vi "ATF-Graph Screen.vi"() -> ()   [LabVIEW 2022 SP3]
panel:
  in  "Monitor":u16=1
  out "Waveform 6":dbl[][](graph)
  out "Waveform 5":waveform(dbl)[](graph)
  out "Waveform 4":waveform(dbl)[](graph)
  out "Waveform 3":waveform(dbl)[](graph)
  out "Waveform 2":waveform(dbl)[](graph)
  out "Waveform 1":waveform(dbl)[](graph)
  in  "EXIT":bool
  # "GRAPH SCREEN"
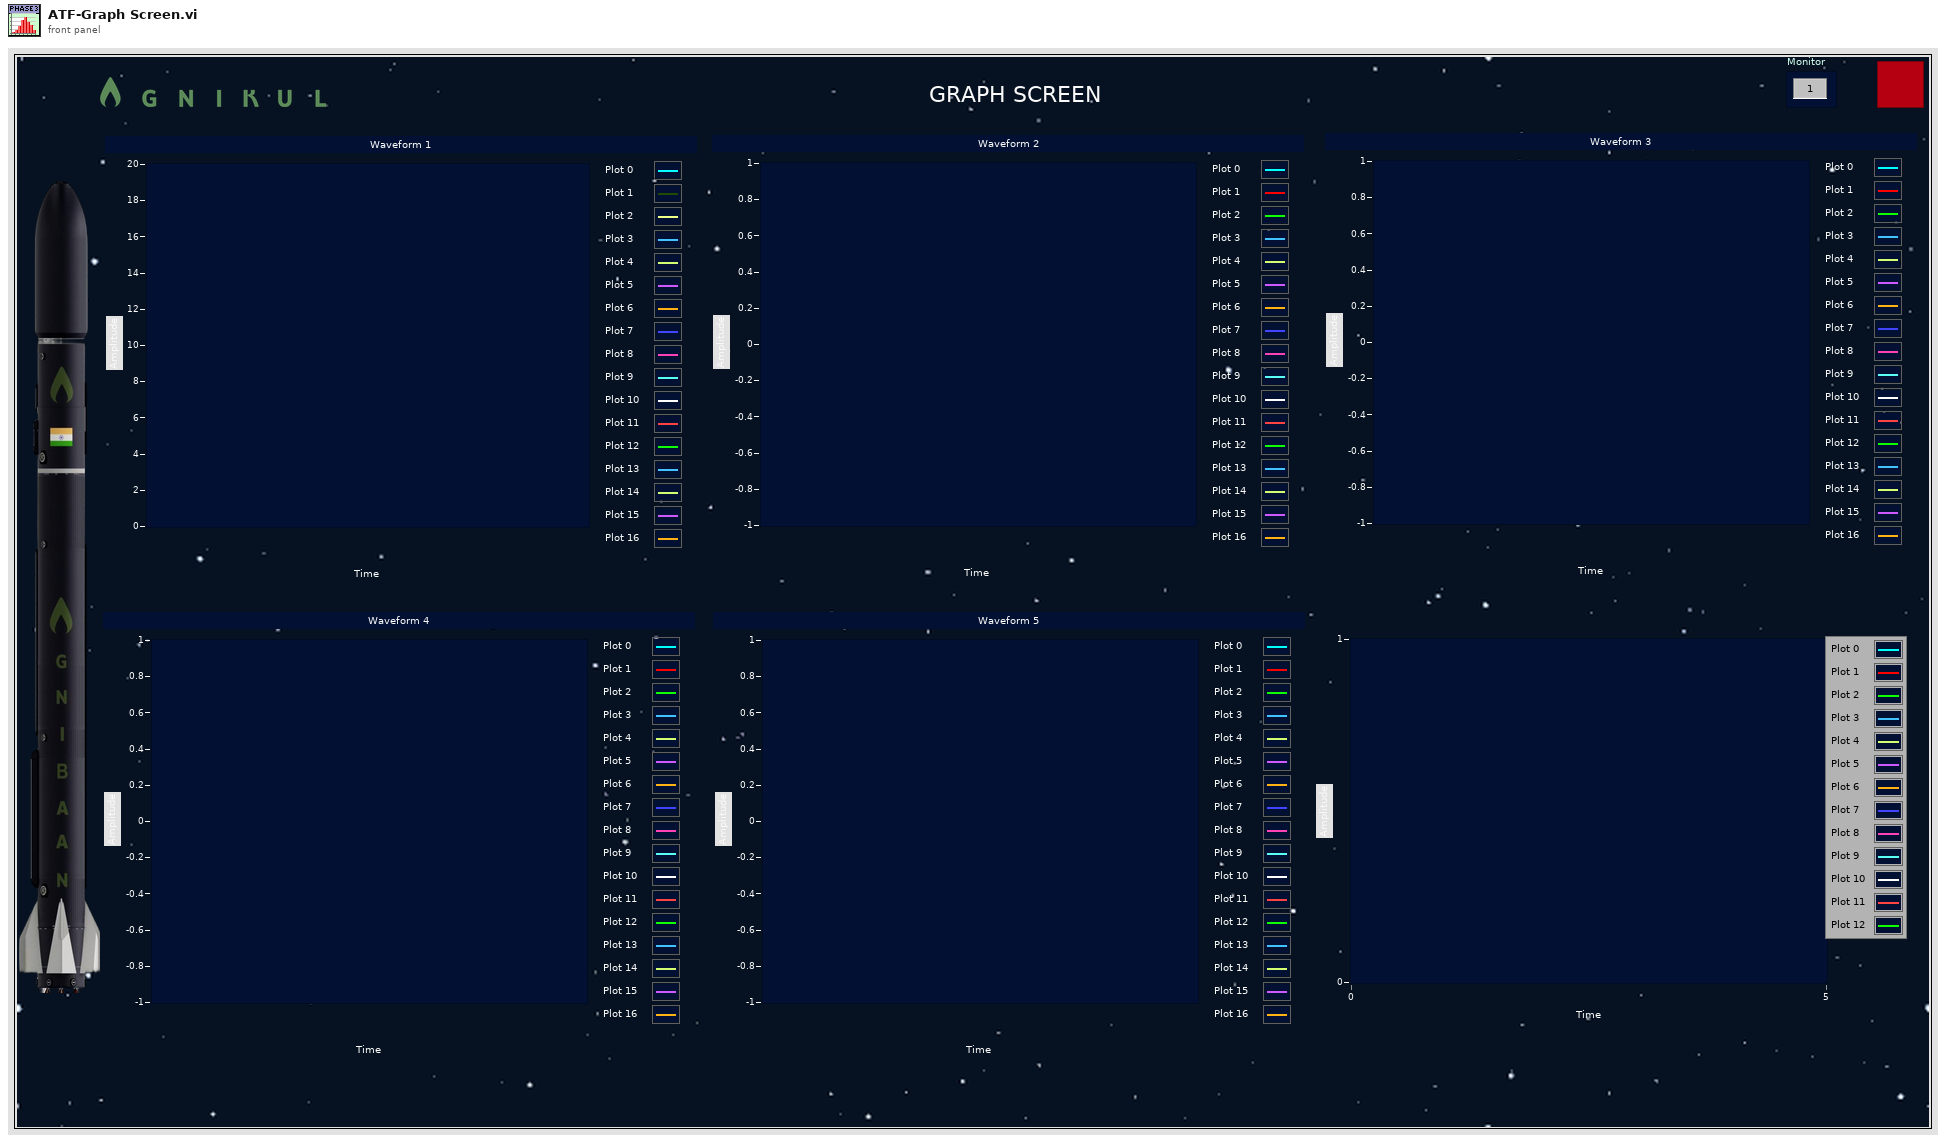
[diagram p1: front panel]
types:
  T1 = enum32{"Invalid", "Standard", "Closed", "Hidden", "Minimized", "Maximized"}
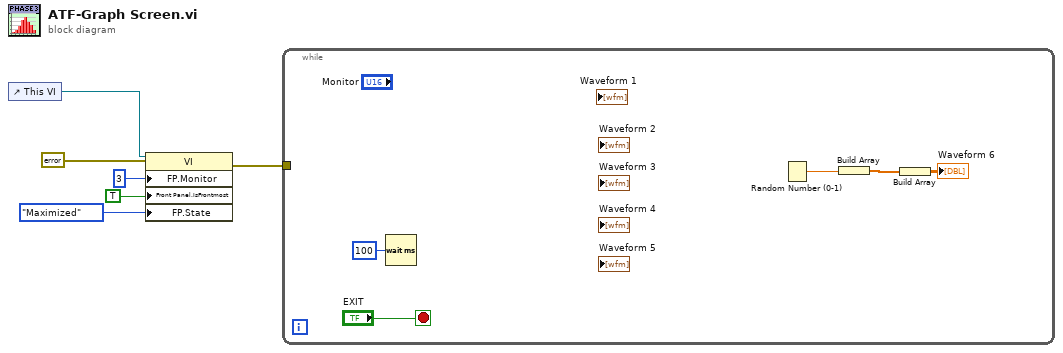
[diagram p0: block diagram]
diagram:
  n1 = control-ref of="This VI"() -> (w6:refnum<vi>)
  n2 = property class="VI"(reference=w6, error in=errorcluster {"status"=FALSE, "code"=0, "source"=""} ("error in (no error)"), "FP.Monitor"=u16 3 ("Front Panel Window:Monitor"), "Front Panel.IsFrontmost"=TRUE ("Front Panel Window:Is Frontmost"), "FP.State"=T1."Maximized" ("Front Panel Window:State")) -> (error out=w2:errorcluster)  [unwired: 1 out]
  n3 = while {
    tunnel: w2 -> [_]
    stop <- "EXIT" stop-if-true
    n4 = Wait (ms)(milliseconds to wait=u32 100) -> ()  [unwired: 1 out]
    n5 = Random Number (0-1)() -> (number: 0 to 1=w9:dbl)
    n6 = Build Array(w9) -> (w8:dbl[])
    n7 = Build Array(w8) -> (→"Waveform 6":dbl[][])
  }
